vi "SetSetpoint.vi"(8 "error in (no error)":errorcluster, 9 "values Q":dbl[](array[numeric]), 10 "values I":dbl[](array[numeric]), 11 "Scope5785_six_channel":refnum<class "Scope5782_six_channel.lvclass">) -> (0 "error out":errorcluster, 3 "Scope5785_six_channel out":refnum<class "Scope5782_six_channel.lvclass">)   [LabVIEW 2018, in "Scope5782_six_channel.lvclass"]
uses:
  Scope5782_six_channel.lvclass
  Scope5782/Scope/controls/Memory block.ctl
  Scope5782_six_channel.lvclass/Scope5782_six_channel.ctl
  FpgaRef/FpgaRef5782/FpgaRef5782.lvclass/FpgaRef5782.ctl
  FpgaRef/FpgaRef5782/FpgaRef5782.lvclass
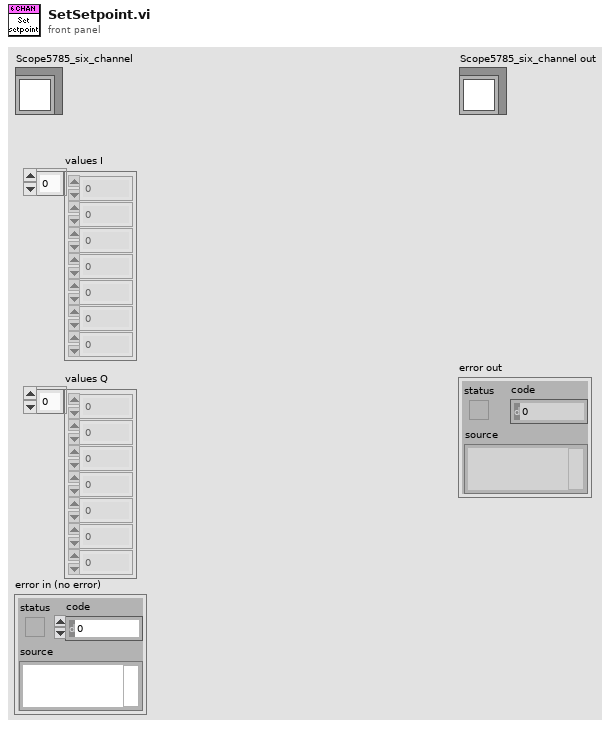
[diagram p1: front panel]
types:
  T1 = typedef "Memory block.ctl" = enum16{"Setpoint", "Beam"}
  T2 = typedef "FPGAref_5782_FeedForward.ctl" = refnum<k20>
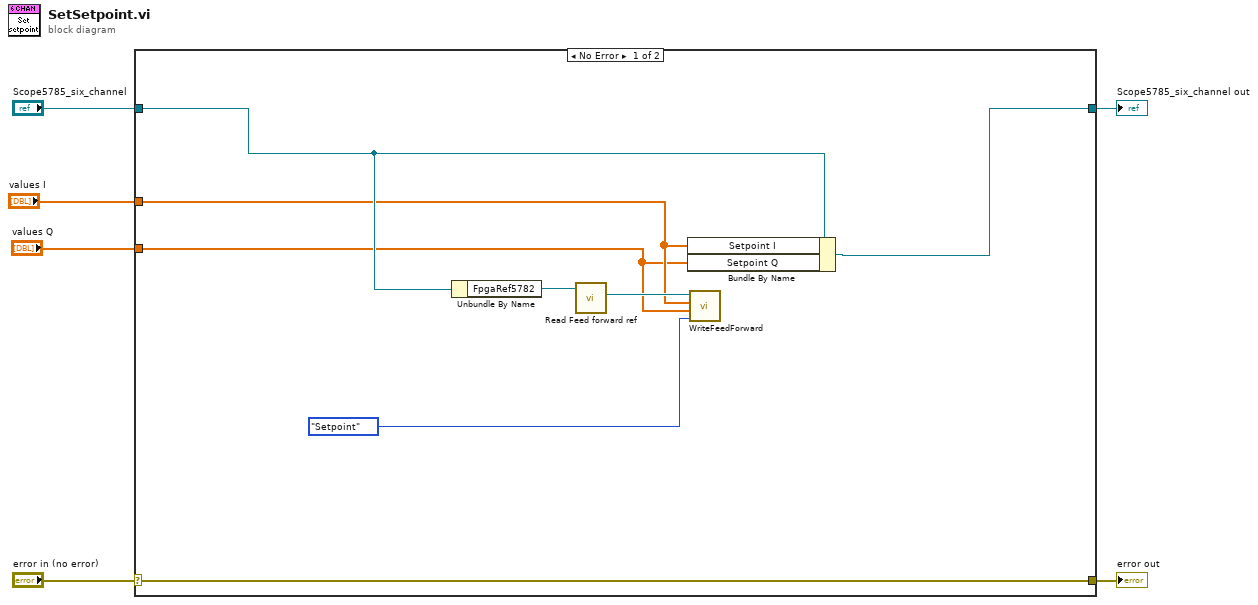
[diagram p0: block diagram]
diagram:
  n1 = case shown="No Error" "error in (no error)" {
    selector: "error in (no error)" -> [w14 w16]
    tunnel: [w14 w16] -> w5
    tunnel: [w9 w15] -> w3
    tunnel: "Scope5785_six_channel" -> [w13 w15]
    tunnel: "values I" -> [w8 _]
    tunnel: "values Q" -> [w7 _]
    frame No Error {
      n2 = Unbundle By Name(w13) -> ("FpgaRef5782"=w12:refnum<class "FpgaRef5782.lvclass">)
      n3 = call "Read Feed forward ref.vi"("FpgaRef5782 in"=w12) -> ("Feed forward ref"=w11:T2)  [unwired: 8 in, 2 out]
      n4 = Bundle By Name(cluster=w13, "Setpoint I"=w8, "Setpoint Q"=w7) -> (w9:refnum<class "Scope5782_six_channel.lvclass">)
      n5 = call "WriteFeedForward.vi"("Memory block"=Memory_block."Setpoint", "values Q"=w7, "values I"=w8, "FPGA VI Reference"=w11) -> ()  [unwired: 7 in, 1 out]
    }
    frame Error {
    }
  }
  "error out" <- w5
  "Scope5785_six_channel out" <- w3
